vi "Substitute Variables.vi"(2 "error in (no error)":errorcluster, 3 "Substitution Rules":T1(array[cluster]), 4 "original formula":string) -> (0 "error out":errorcluster, 1 "formula after substitution":string)   [LabVIEW 2009]
doc: "Substitutes a formula string by given rules. The rules have a <B>parameter name</B> - <B>parameter content</B> structure."
panel:
  # "Example:\n\n original formula: A*x+B^2 \n Substitution Rules: \n   A and sin(x)\n   B and cos(x)"
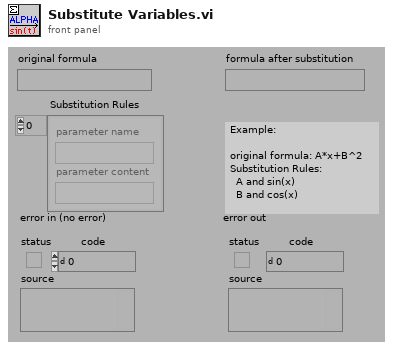
[diagram p1: front panel]
types:
  T1 = cluster{"parameter name":string, "parameter content":string}[]
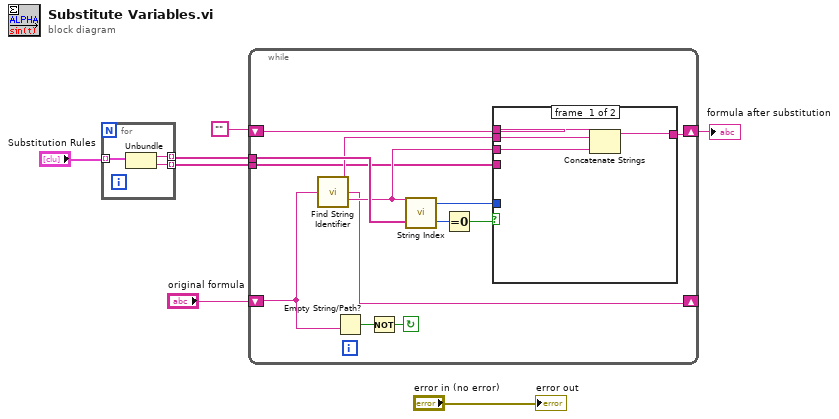
[diagram p0: block diagram]
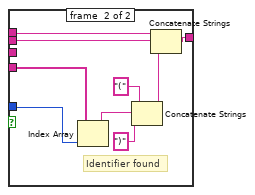
[diagram p2: hidden frame]
diagram:
  n1 = for {
    tunnel: "Substitution Rules" -> [w10] mode=indexing
    tunnel: [w9] -> w3 mode=indexing
    tunnel: [w8] -> w2 mode=indexing
    n2 = Unbundle(w10) -> ("parameter name"=w9:string, "parameter content"=w8:string)
  }
  n3 = while {
    tunnel: w2 -> [w12]
    shift-left: "" -> [w16]
    shift-right: [w17] -> w5
    shift-left: "original formula" -> [w21]
    shift-right: [w11] -> _
    tunnel: w3 -> [w15]
    stop <- w22 continue-if-true
    n4 = call "Find String Identifier.vi"("input string"=w21) -> ("before string"=w14:string, "remaining string"=w11:string, "identifier"=w13:string)
    n5 = Empty String/Path?(string/path=w21) -> (empty?=w23:bool)
    n6 = Not(x=w23) -> (.not. x?=w22:bool)
    n7 = call "String Index.vi"("String Array"=w15, "search string"=w13) -> ("error"=w19:i32, "index"=w18:i32)
    n8 = Equal To 0?(x=w19) -> (x = 0?=w20:bool)
    n9 = case shown="True" w20 {
      tunnel: w18 -> [_ w34]
      tunnel: w16 -> [w26 w31]
      tunnel: [w27 w32] -> w17
      tunnel: w14 -> [w25 w30]
      tunnel: w13 -> [w24 _]
      tunnel: w12 -> [_ w28]
      frame #0 {
        n10 = Concatenate Strings(w26, w25, w24) -> (w27:string)
      }
      frame #1 {
        # "Identifier found"
        n11 = Index Array(array=w28, index=w34) -> (element=w33:string)
        n12 = Concatenate Strings("(", w33, ")") -> (w29:string)
        n13 = Concatenate Strings(w31, w30, w29) -> (w32:string)
      }
    }
  }
  "formula after substitution" <- w5
  "error out" <- "error in (no error)"
